vi "FTW-Supervisor-LogEvent.vi"(0 "FTW Supervisor Connection":refnum<class "FTW-Supervisor-Connector.lvclass">, 5 "Event Type":string, 7 "Event Data":string, 9 "Source (unwired for call chain)":string="CallChain", 11 "error in":errorcluster) -> (4 "FTW Supervisor Connection out":refnum<class "FTW-Supervisor-Connector.lvclass">, 15 "error out":errorcluster)   [LabVIEW 2014, in "FTW-Supervisor-Connector.lvclass"]
uses:
  FTW-Supervisor-Connector.lvclass
  codegen/xnode/FTW-Actor-Ask.xnode
  socket/connector/core/FTW-Connector-Core-Type.ctl
  time/FTW-Time-RelativeTimer.vi
  socket/support/FTW-Socket-Core-LibraryError.vi
  lib/FTW-KernelFilepath.vi
  codegen/xnode/FTW-JSON-Fetch.xnode
  request/FTW-Request-InterpretResponse.vi
  error/FTW-ERR-ThrowError.vi
  codegen/xnode/json/fetch/FTW-JSON-Core-GetFlattenedValue.vi
  reflection/FTW-Reflection-Type.vi
  json/core/FTW-JSON-Core-EncodingFlags.vi
  error/FTW-ERR-NoErrorConstant.vi
panel:
  # "Inputs"
  # "Outputs"
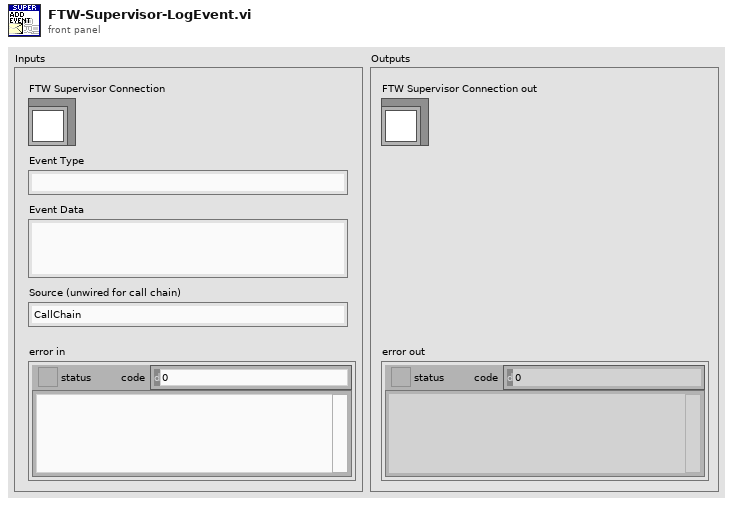
[diagram p1: front panel]
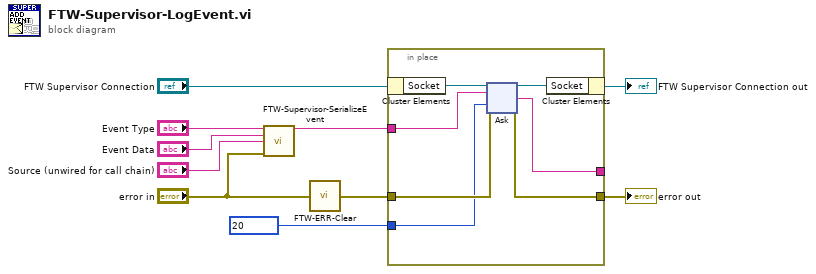
[diagram p0: block diagram]
diagram:
  n1 = call "FTW-Supervisor-SerializeEvent.vi"("Event Type"="Event Type", "Event Data"="Event Data", "Source"="Source (unwired for call chain)", "Error to Log"="error in") -> ("Serialized Event"=w3:string)  [unwired: 11 in]
  n2 = call "FTW-ERR-Clear.vi"("error to snuff"="error in") -> ("no error"=w4:errorcluster)
  n3 = in-place {
    in-place-border: w4 -> [w13]
    in-place-border: [w17] -> w1
    in-place-border: [w14] -> _
    in-place-border: w3 -> [w12]
    in-place-border: 20 ("Receive Timeout") -> [w11]
    n4 = in-place-cluster #1("FTW Supervisor Connection") -> ("Socket"=w16:refnum<data-value>)
    n5 = xnode "Ask"("FTW Actor Connector"=w16, "Request"=w12, "Timeout"=w11, "error in"=w13) -> ("FTW Actor Connector out"=w15:refnum<data-value>, "Response"=w14:string, "error out"=w17:errorcluster)  [unwired: 1 in, 1 out]
    n6 = in-place-cluster #1("Socket"=w15) -> (→"FTW Supervisor Connection out":refnum<class "FTW-Supervisor-Connector.lvclass">)
  }
  "error out" <- w1
